vi "Set_Arguments.vi"(8 "error in (no error)":errorcluster caption="entrée d'erreur (pas d'erreur)", 10 "Arguments":string, 11 "Flash_Jlink en entrée":refnum<class "Flash_AVRDUDE.lvclass">) -> (0 "error out":errorcluster caption="sortie d'erreur", 3 "Flash_Jlink en sortie":refnum<class "Flash_AVRDUDE.lvclass">)   [LabVIEW 2020, in "Library Test.lvlib" / "Flash_AVRDUDE.lvclass"]
uses:
  Flash_AVRDUDE.lvclass
  Flash_AVRDUDE.lvclass/Flash_AVRDUDE.ctl
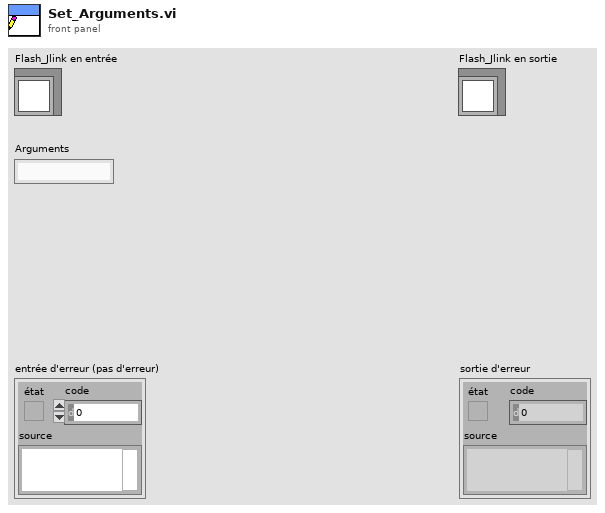
[diagram p1: front panel]
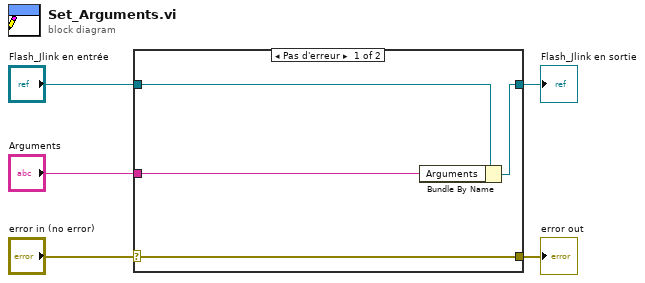
[diagram p0: block diagram]
diagram:
  n1 = case shown="Pas d'erreur" "error in (no error)" {
    selector: "error in (no error)" -> [w9 w10]
    tunnel: [w9 w10] -> w4
    tunnel: [w7 w11] -> w2
    tunnel: "Flash_Jlink en entrée" -> [w8 w11]
    tunnel: "Arguments" -> [w6 _]
    frame No Error {
      n2 = Bundle By Name(cluster=w8, "Arguments"=w6) -> (w7:refnum<class "Flash_AVRDUDE.lvclass">)
    }
    frame Error {
    }
  }
  "error out" <- w4
  "Flash_Jlink en sortie" <- w2
